vi "PCTrig.vi"(0 "object in":refnum<class "AD2_SDK.lvclass">, 5 "error in (no error)":errorcluster) -> (14 "object out":refnum<class "AD2_SDK.lvclass">, 19 "error out":errorcluster)   [LabVIEW 2021, in "AD2_SDK.lvclass"]
uses:
  AD2_SDK.lvclass
  AD2_SDK.lvclass/AD2_SDK.ctl
  Olasdwf/Olasdwf.lvlib
panel:
  out "function return":i32
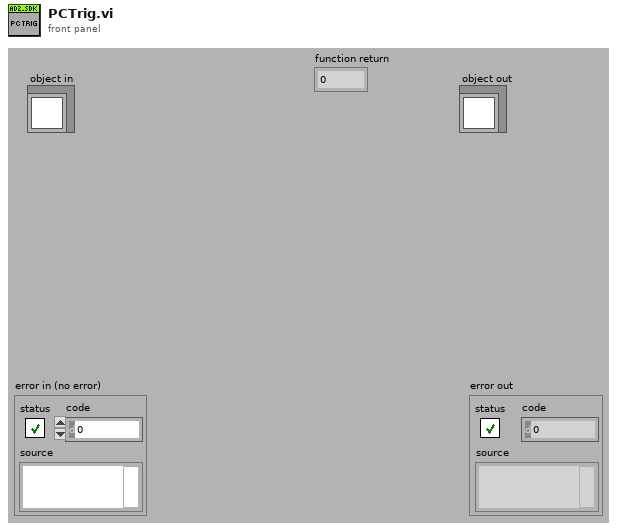
[diagram p1: front panel]
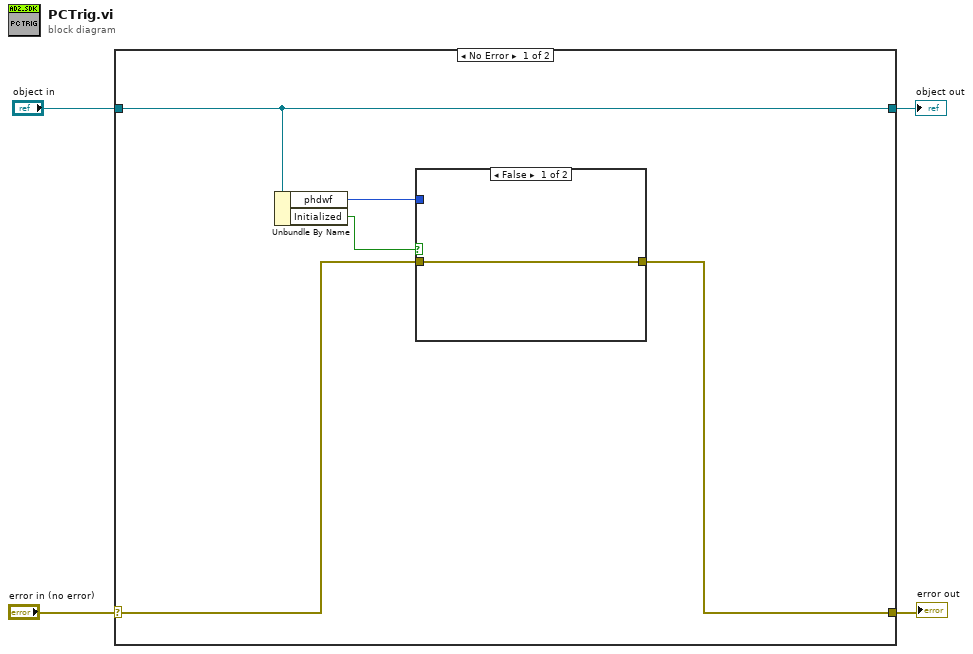
[diagram p0: block diagram]
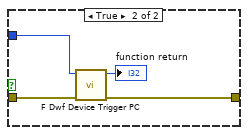
[diagram p2: hidden frame]
diagram:
  n1 = case shown="No Error" "error in (no error)" {
    selector: "error in (no error)" -> [w7 w16]
    tunnel: [w6 w16] -> w3
    tunnel: [w9 w15] -> w1
    tunnel: "object in" -> [w9 w15]
    frame No Error {
      n2 = Unbundle By Name(w9) -> ("phdwf"=w8:i32, "Initialized"=w5:bool)
      n3 = case shown="False" w5 {
        tunnel: w8 -> [_ w14]
        tunnel: w7 -> [w10 w13]
        tunnel: [w10 w12] -> w6
        frame False {
        }
        frame True {
          n4 = call "F Dwf Device Trigger PC.vi"("error in (no error)"=w13, "hdwf"=w14) -> ("error out"=w12:errorcluster, "function return"=→"function return":i32)  [unwired: 8 in]
        }
      }
    }
    frame Error {
    }
  }
  "error out" <- w3
  "object out" <- w1
